vi "(SubVI)Launcher_Get HTTP Header Field Value.vi"(0 "client handle in":T1 caption="클라이언트 핸들 출력", 5 "Header in":string, 7 "Field":string, 11 "error in (no error)":errorcluster caption="에러 입력(에러 없음)") -> (4 "client handle out":T1 caption="클라이언트 핸들 출력", 6 "Header out":string, 8 "Value":string, 10 "Found?":bool, 15 "error out":errorcluster caption="에러 출력")   [LabVIEW 2020]
uses:
  <vilib>/httpClient/ClientHandle.ctl
  <vilib>/httpClient/LabVIEWHTTPClient.lvlib
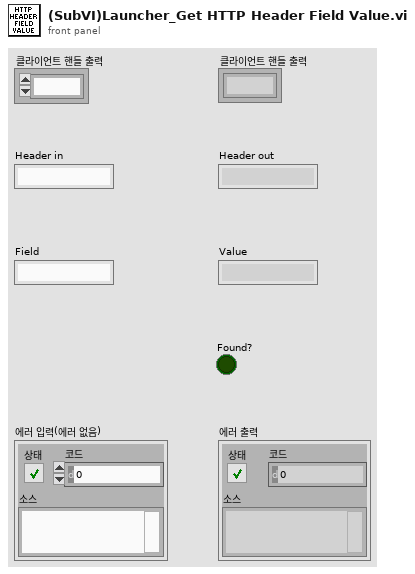
[diagram p1: front panel]
types:
  T1 = typedef "LabVIEWHTTPClient.lvlib/ClientHandle.ctl" = refnum<k1>
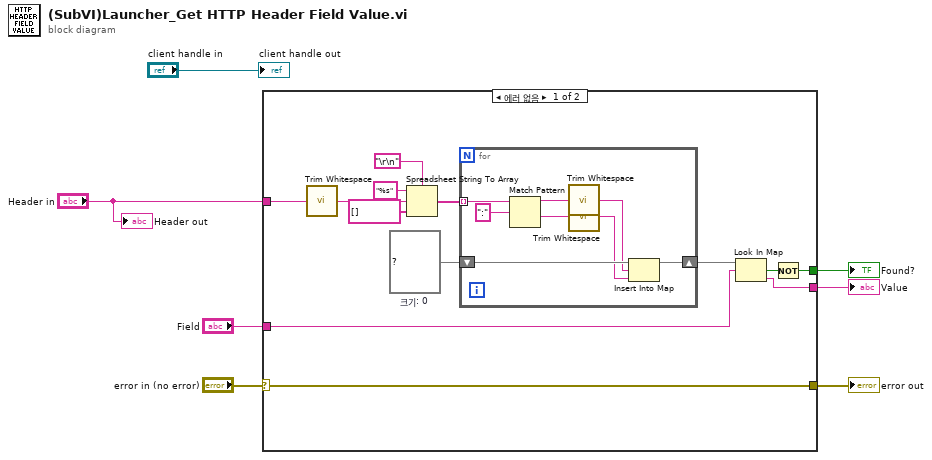
[diagram p0: block diagram]
diagram:
  n1 = case shown="에러 없음" "error in (no error)" {
    selector: "error in (no error)" -> [w13 w29]
    tunnel: [w13 w29] -> w6
    tunnel: "Header in" -> [w12 _]
    tunnel: [w8 _] -> w4
    tunnel: [w10 _] -> w3
    tunnel: "Field" -> [w9 _]
    frame No Error {
      w19 = map{string, string} {}  # 크기: 0
      n2 = call <vilib>:"Trim Whitespace.vi"("string"=w12) -> ("trimmed string"=w18:string)  [unwired: 1 in]
      n3 = Spreadsheet String To Array(delimiter (Tab)="\r\n" ("구분 문자 (탭)"), format string="%s" ("포맷 문자열"), spreadsheet string=w18, array type (2D Dbl)=string[] []) -> (array=w17:string[])
      n4 = for {
        tunnel: w17 -> [w27] mode=indexing
        shift-right: [w21] -> w20
        shift-left: w19 -> [w24]
        n5 = Match Pattern(string=w27, regular expression=":" ("포맷 문자열")) -> (before substring=w28:string, after substring=w25:string)  [unwired: 1 in, 2 out]
        n6 = call <vilib>:"Trim Whitespace.vi"("string"=w28) -> ("trimmed string"=w23:string)  [unwired: 1 in]
        n7 = call <vilib>:"Trim Whitespace.vi"("string"=w25) -> ("trimmed string"=w22:string)  [unwired: 1 in]
        n8 = Insert Into Map(map in=w24, key=w23, value=w22) -> (map out=w21:map{string, string})  [unwired: 2 out]
      }
      n9 = Look In Map(map=w20, key=w9) -> (key not found?=w11:bool, value=w10:string)  [unwired: 1 in]
      n10 = Not(x=w11) -> (.not. x?=w8:bool)
    }
    frame Error {
    }
  }
  "error out" <- w6
  "Value" <- w3
  "Found?" <- w4
  "Header out" <- "Header in"
  "client handle out" <- "client handle in"
